vi "RT Driver VI.vi"(7 "Operation":T1, 11 "Device Reference in":T2 format="%.0x") -> (0 "Error Code":i32)   [LabVIEW 2019, in "OPC UA Client Addon Engine.lvlib"]
uses:
  OPC UA Client Addon Engine.lvlib
  <vilib>/NI VeriStand/Custom Device API/Data Reference.ctl
  <vilib>/NI VeriStand/Custom Device API/Custom Device API.lvlib
  Addon Shared/OPCConnection.Properties.ctl
  Addon Shared/OPC UA Client Addon Shared.lvlib
  Addon Shared/Compiled.Settings.ctl
  Addon Shared/Poll.ListProperties.ctl
  Types/Poll.Parameters.ctl
  Types/Main.StateVariables.ctl
  Addon Shared/Tag.WriteProperties.Info.ctl
  Addon Shared/Tags.ReadWriteRefs.ctl
  <vilib>/NI VeriStand/Custom Device API/Custom Device Target Type.ctl
  <vilib>/NI/NIVS Inline Async API/_VS Inline Async API/VS Inline Async API/VS Inline Async API.lvclass
  <vilib>/NI/NIVS Inline Async API/_VS Inline Async API/VS Inline Async API/Types/Error Handling Settings.ctl
  <vilib>/NI VeriStand/Custom Device API/Custom Device Item Ref.ctl
  <vilib>/NI VeriStand/Custom Device API/Hardware Interface Driver VI Operation.ctl
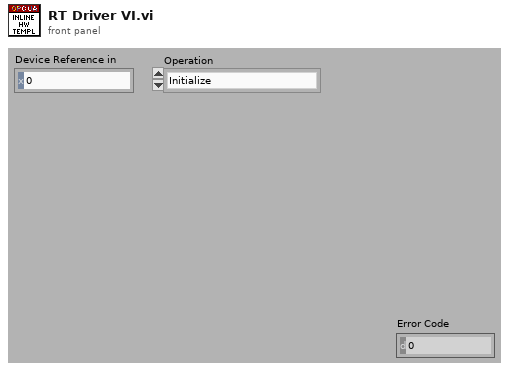
[diagram p1: front panel]
types:
  T1 = typedef "Custom Device API.lvlib/Hardware Interface Driver VI Operation.ctl" = enum16{"Initialize", "Start", "Read Data from HW", "Write Data to HW", "Close"}
  T2 = typedef "Custom Device API.lvlib/Custom Device Item Ref.ctl" = u64
  T3 = typedef "OPC UA Client Addon Engine.lvlib/Main.StateVariables.ctl" = cluster{"Parameters":T4, "Processes":refnum<class "VS Inline Async API.lvclass">}
  T4 = typedef "OPC UA Client Addon Engine.lvlib/Poll.Parameters.ctl" = cluster{"Name":string, "Settings":T5, "WriteData":refnum<k33>, "ReadData":refnum<k33>, "WriteUpdate":refnum<k33>, "ReadUpdate":refnum<k33>}
  T5 = typedef "OPC UA Client Addon Shared.lvlib/Compiled.Settings.ctl" = cluster{"Connection.Properties":T6, "PollEngine.Settings":T7[], "LUT":variant, "Write Locations":T8[], "TotalTags":u32, "Data Refs":T9, "Target Type":T11}
  T6 = typedef "OPC UA Client Addon Shared.lvlib/OPCConnection.Properties.ctl" = cluster{"Server IP Address":string, "Server Port":u16, "Message Mode":enum16{"None", "Sign", "Sign and Encrypt"}, "Security":enum16{"Basic256", "Basic128Rsa15"}, "User Name":string, "Password":string, "Client Certificate":path, "Server Certificate":path, "Server Certificate (RT)":path, "Client Certificate (RT)":path}
  T7 = typedef "OPC UA Client Addon Shared.lvlib/Poll.ListProperties.ctl" = cluster{"Poll Rate":dbl, "Tags":string[]}
  T8 = typedef "OPC UA Client Addon Shared.lvlib/Tag.WriteProperties.Info.ctl" = cluster{"Path":string, "Offset":i32, "Length":i32, "DataType":u32}
  T9 = typedef "OPC UA Client Addon Shared.lvlib/Tags.ReadWriteRefs.ctl" = cluster{"Read Refs":T10[], "Read Values":dbl[], "Read?":bool[], "Access":enum8{"Null", "Read", "Write", "Read&Write"}[], "Write Refs":T10[], "Write Values":dbl[], "Write?":bool[], "Write Only Location":u32, "Write? Reset":bool[]}
  T10 = typedef "Custom Device API.lvlib/Data Reference.ctl" = i32
  T11 = typedef "Custom Device API.lvlib/Custom Device Target Type.ctl" = enum16{"PharLap", "VxWorks", "Windows", "Linux_32_ARM", "Linux_x64"}
  T12 = typedef "VS Inline Async API.lvlib/VS Inline Async API.lvclass/Error Handling Settings.ctl" = cluster{"Write to SystemLog (F)":bool}
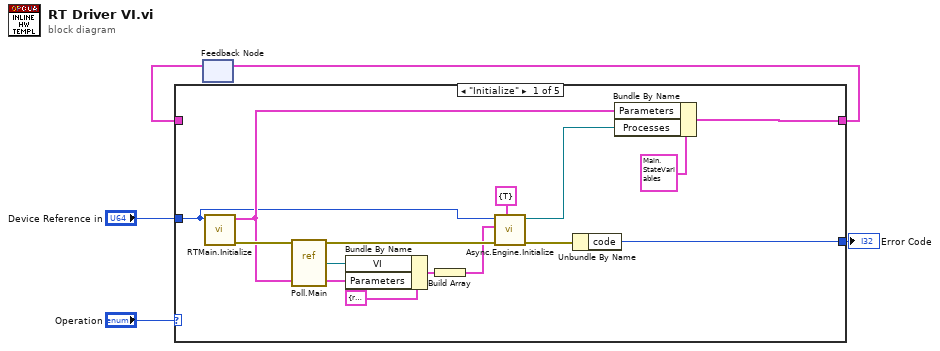
[diagram p0: block diagram]
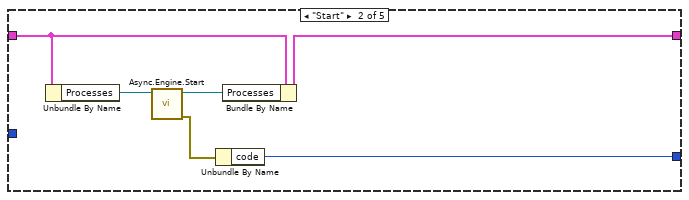
[diagram p2: hidden frame]
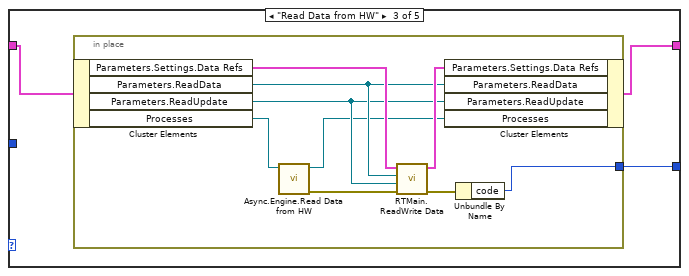
[diagram p3: hidden frame]
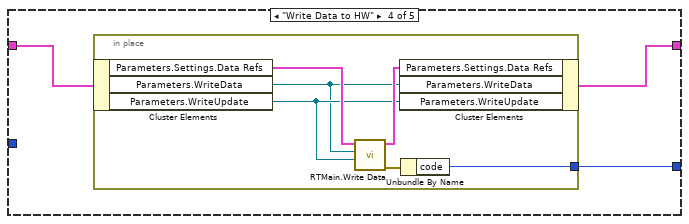
[diagram p4: hidden frame]
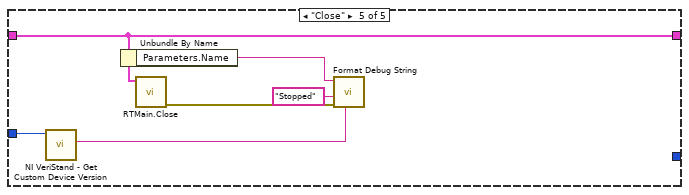
[diagram p5: hidden frame]
diagram:
  n1 = feedback #1() -> (w3:T3)  [unwired: 1 out]
  n2 = case shown="\"Initialize\"" "Operation" {
    tunnel: [w17 w22 w25 w37 w47] -> w4
    tunnel: w3 -> [_ w23 w26 w38 w47]
    tunnel: "Device Reference in" -> [w9 _ _ _ w51]
    tunnel: [w18 w24 w27 w39 _] -> w1
    frame "Initialize" {
      n3 = call "RTMain.Initialize.vi"("Device Reference in"=w9) -> ("error out"=w15:errorcluster, "Parameters"=w12:T4)  [unwired: 8 in, 1 out]
      n4 = vi-ref "Poll.Main.vi"() -> (w13:refnum<vi>)
      n5 = Bundle By Name(cluster=cluster{"VI":refnum<vi>, "Parameters":variant} {"VI"=refnum, "Parameters"=variant} ("Process"), "VI"=w13, "Parameters"=w12) -> (w11:cluster{"VI":refnum<vi>, "Parameters":variant})
      n6 = Build Array(w11) -> (w10:cluster{"VI":refnum<vi>, "Parameters":variant}[])
      n7 = call <vilib>:"Async.Engine.Initialize.vi"("Error Log Settings"=T12 {"Write to SystemLog (F)"=TRUE}, "error in (no error)"=w15, "Processes"=w10, "Custom Device Ref"=w9) -> ("error out"=w8:errorcluster, "Async"=w7:refnum<class "VS Inline Async API.lvclass">)  [unwired: 6 in]
      n8 = Unbundle By Name(w8) -> ("code"=w18:i32)
      n9 = Bundle By Name(cluster=T3 {"Parameters"={"Name"="", "Settings"={"Connection.Properties"={"Server IP Address"="", "Server Port"=0, "Message Mode"=enum."None", "Security"=enum."Basic256", "User Name"="", "Password"="", "Client Certificate"=path "", "Server Certificate"=path "", "Server Certificate (RT)"=path "", "Client Certificate (RT)"=path ""}, "PollEngine.Settings"=[], "LUT"=variant, "Write Locations"=[], "TotalTags"=0, "Data Refs"={"Read Refs"=[], "Read Values"=[], "Read?"=[], "Access"=[], "Write Refs"=[], "Write Values"=[], "Write?"=[], "Write Only Location"=0, "Write? Reset"=[]}, "Target Type"=enum."PharLap"}, "WriteData"=refnum, "ReadData"=refnum, "WriteUpdate"=refnum, "ReadUpdate"=refnum}, "Processes"=refnum}, "Parameters"=w12, "Processes"=w7) -> (w17:T3)
    }
    frame "Start" {
      n10 = Unbundle By Name(w23) -> ("Processes"=w21:refnum<class "VS Inline Async API.lvclass">)
      n11 = call <vilib>:"Async.Engine.Start.vi"("VS Inline Async API in"=w21) -> ("error out"=w19:errorcluster, "VS Inline Async API out"=w20:refnum<class "VS Inline Async API.lvclass">)  [unwired: 9 in]
      n12 = Unbundle By Name(w19) -> ("code"=w24:i32)
      n13 = Bundle By Name(cluster=w23, "Processes"=w20) -> (w22:T3)
    }
    frame "Read Data from HW" {
      n14 = in-place {
        in-place-border: [w36] -> w27
        n15 = in-place-cluster #2(w26) -> ("Parameters.Settings.Data Refs"=w33:T9, "Parameters.ReadData"=w30:refnum<k33>, "Parameters.ReadUpdate"=w29:refnum<k33>, "Processes"=w31:refnum<class "VS Inline Async API.lvclass">)
        n16 = call <vilib>:"Async.Engine.Read Data from HW.vi"("Async in"=w31) -> ("error out"=w35:errorcluster, "Async out"=w28:refnum<class "VS Inline Async API.lvclass">)  [unwired: 9 in]
        n17 = call "RTMain.ReadWrite Data.vi"("error in"=w35, "ReadUpdate"=w29, "Write to VS Engine FIFO"=w30, "Data Refs"=w33) -> ("error out"=w34:errorcluster, "Data Refs"=w32:T9)  [unwired: 5 in, 1 out]
        n18 = in-place-cluster #2("Parameters.Settings.Data Refs"=w32, "Parameters.ReadData"=w30, "Parameters.ReadUpdate"=w29, "Processes"=w28) -> (w25:T3)
        n19 = Unbundle By Name(w34) -> ("code"=w36:i32)
      }
    }
    frame "Write Data to HW" {
      n20 = in-place {
        in-place-border: [w45] -> w39
        n21 = in-place-cluster #3(w38) -> ("Parameters.Settings.Data Refs"=w43:T9, "Parameters.WriteData"=w40:refnum<k33>, "Parameters.WriteUpdate"=w41:refnum<k33>)
        n22 = call "RTMain.Write Data.vi"("WriteUpdate"=w41, "Read from VS Engine FIFO"=w40, "Data Refs"=w43) -> ("error out"=w44:errorcluster, "Data Refs"=w42:T9)  [unwired: 7 in]
        n23 = in-place-cluster #3("Parameters.Settings.Data Refs"=w42, "Parameters.WriteData"=w40, "Parameters.WriteUpdate"=w41) -> (w37:T3)
        n24 = Unbundle By Name(w44) -> ("code"=w45:i32)
      }
    }
    frame "Close" {
      n25 = call <vilib>:"NI VeriStand - Get Custom Device Version.vi"("Device Ref in"=w51) -> ("Value"=w49:string)  [unwired: 8 in, 2 out]
      n26 = Unbundle By Name(w47) -> ("Parameters.Name"=w46:string)
      n27 = call "RTMain.Close.vi"("cluster"=w47) -> ("error out"=w48:errorcluster)  [unwired: 10 in]
      n28 = call "Format Debug String.vi"("Version"=w49, "error in (no error)"=w48, "State"="Stopped", "Name"=w46) -> ()  [unwired: 7 in, 1 out]
    }
  }
  "Error Code" <- w1
  n29 = feedback-in #1(w4) -> ()
